vi "C867_Get_Answer.vi"(8 "entrée d'erreur (pas d'erreur)":errorcluster, 11 "ID en entrée":i32) -> (0 "sortie d'erreur":errorcluster, 1 "BOOL":i32, 2 "szAnswer":string, 3 "ID en sortie":i32)   [LabVIEW 2026]
uses:
  C867-VIs/Low Level/PI_GCS2_DLL_x64.dll
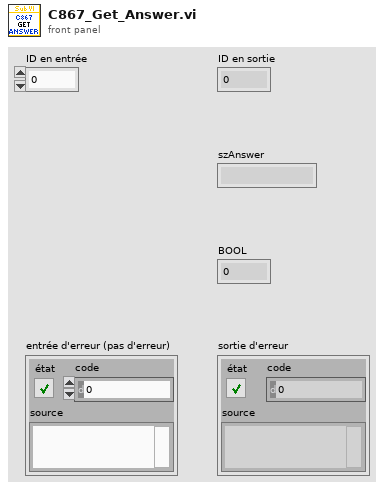
[diagram p1: front panel]
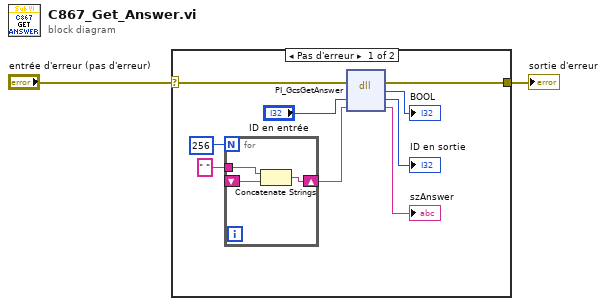
[diagram p0: block diagram]
diagram:
  n1 = case shown="Pas d'erreur" "entrée d'erreur (pas d'erreur)" {
    selector: "entrée d'erreur (pas d'erreur)" -> [w8 w15]
    tunnel: [w11 w15] -> w2
    frame No Error {
      n2 = for {
        N: 256 -> [_]
        tunnel: " " -> [w14]
        shift-right: [w13] -> w3
        shift-left: _ -> [w12]
        n3 = Concatenate Strings(w14, w12) -> (w13:string)
      }
      n4 = dll-call lib="D:/SEBASTIEN/GitHub/LABVIEW-Useful-codes/Device_control/PC-C867-IO Control/v0.2/SubVI/PI-C867/C867-VIs/Low Level/PI_GCS2_DLL_x64.dll" fn="PI_GcsGetAnswer"(error in=w8, "ID"="ID en entrée", "szAnswer"=w3) -> (error out=w11:errorcluster, "BOOL"=→"BOOL":i32, "ID"=→"ID en sortie":i32, "szAnswer"=→"szAnswer":string)  [unwired: 2 in, 1 out]
    }
    frame Error {
    }
  }
  "sortie d'erreur" <- w2
